vi "AddConfigurationFiles.vi"(6 "path root vi ref (calling vi)":refnum<vi>, 8 "error in (no error)":errorcluster, 10 "configuration files":path[](array[path]), 11 "VeriStandTestCase in":refnum<class "VeriStandTestCase.lvclass">) -> (0 "error out":errorcluster, 3 "VeriStandTestCase out":refnum<class "VeriStandTestCase.lvclass">)   [LabVIEW 2016, in "VeriStandTestCase.lvclass"]
uses:
  VeriStandTestCase.lvclass
  VeriStandTestCase.lvclass/VeriStandTestCase.ctl
  VeriStandTestUtilities/VeriStandTestUtilities.lvlib
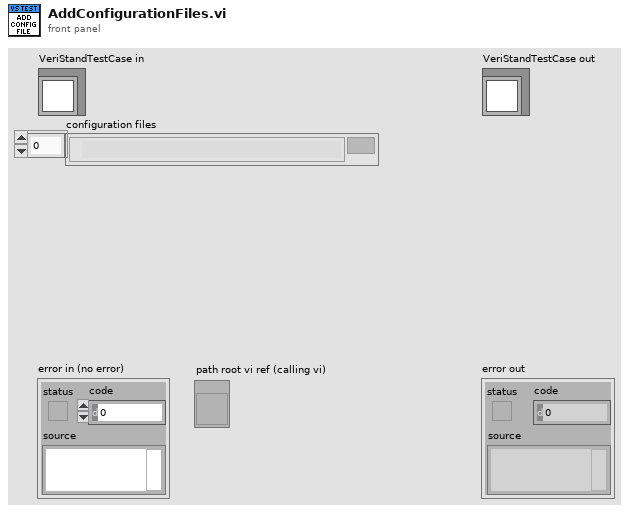
[diagram p1: front panel]
types:
  T1 = typedef "VeriStandTestUtilities.lvlib/ConfigPropertyItem.ctl" = cluster{"key":string, "value":string}
  T2 = typedef "VeriStandTestUtilities.lvlib/ConfigOverrideItem.ctl" = cluster{"node":string, "property":string, "value":string}
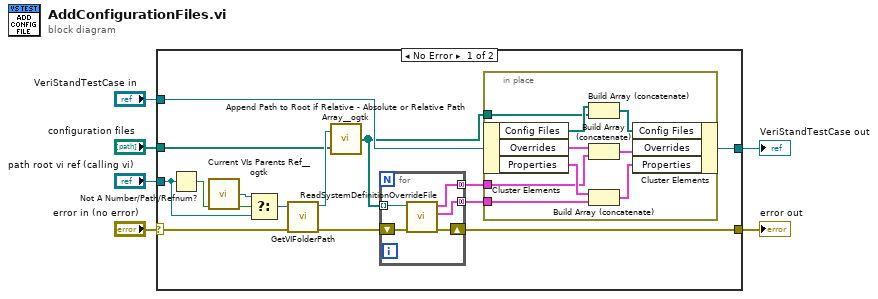
[diagram p0: block diagram]
diagram:
  n1 = case shown="No Error" "error in (no error)" {
    selector: "error in (no error)" -> [w16 w36]
    tunnel: [w8 w36] -> w5
    tunnel: [w19 w35] -> w3
    tunnel: "VeriStandTestCase in" -> [w20 w35]
    tunnel: "configuration files" -> [w17 _]
    tunnel: "path root vi ref (calling vi)" -> [w7 _]
    frame No Error {
      n2 = Not A Number/Path/Refnum?(number/path/refnum=w7) -> (NaN/Path/Refnum?=w15:bool)
      n3 = call <userlib>:"Current VIs Parents Ref__ogtk.vi"() -> ("Calling VI's Reference"=w14:refnum<vi>)  [unwired: 2 in]
      n4 = Select(t=w14, s=w15, f=w7) -> (s? t:f=w13:refnum<vi>)
      n5 = call "GetVIFolderPath.vi"("error in (no error)"=w16, "VI Reference in"=w13) -> ("error out"=w9:errorcluster, "VI Folder Path out"=w18:path)  [unwired: 8 in]
      n6 = call <userlib>:"Append Path to Root if Relative - Absolute or Relative Path Array__ogtk.vi"("Absolute or Relative Paths"=w17, "Root Path"=w18) -> ("Absolute or Appended Paths"=w12:path[])
      n7 = for {
        shift-right: [w33] -> w8
        shift-left: w9 -> [w34]
        tunnel: w12 -> [w32] mode=indexing
        tunnel: [w31] -> w10 mode=concatenating
        tunnel: [w30] -> w11 mode=concatenating
        n8 = call "ReadSystemDefinitionOverrideFile.vi"("error in (no error)"=w34, "configuration file path"=w32) -> ("error out"=w33:errorcluster, "properties"=w30:T1[], "overrides"=w31:T2[])  [unwired: 7 in]
      }
      n9 = in-place {
        in-place-border: w12 -> [w27]
        in-place-border: w11 -> [w26]
        in-place-border: w10 -> [w21]
        n10 = in-place-cluster #1(w20) -> ("Config Files"=w29:path[], "Overrides"=w23:T2[], "Properties"=w24:T1[])
        n11 = Build Array (concatenate)(w29, w27) -> (w28:path[])
        n12 = Build Array (concatenate)(w23, w21) -> (w22:T2[])
        n13 = Build Array (concatenate)(w24, w26) -> (w25:T1[])
        n14 = in-place-cluster #1("Config Files"=w28, "Overrides"=w22, "Properties"=w25) -> (w19:refnum<class "VeriStandTestCase.lvclass">)
      }
    }
    frame Error {
    }
  }
  "error out" <- w5
  "VeriStandTestCase out" <- w3
